vi "Unintentional Island Occurence.vi"(8 "error in":errorcluster, 10 "Unintentional Island":bool, 11 "SCADA in":refnum<class "EMS.lvclass">) -> (0 "error out":errorcluster, 3 "SCADA out":refnum<class "EMS.lvclass">)   [LabVIEW 2018, in "EMS Core.lvlib" / "EMS.lvclass"]
uses:
  EMS.lvclass
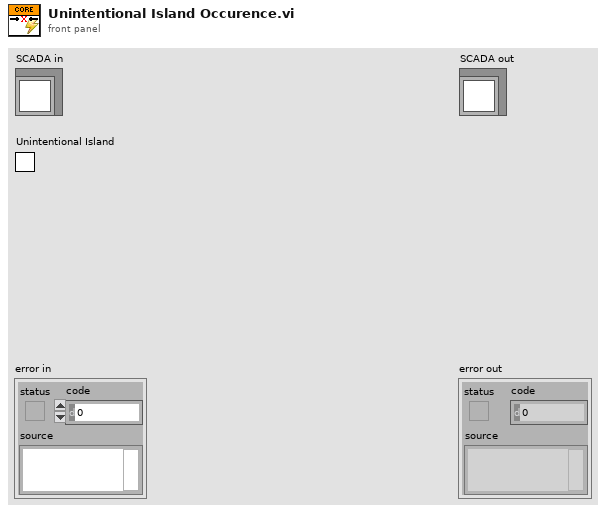
[diagram p1: front panel]
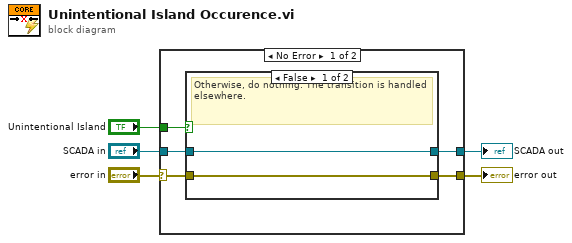
[diagram p0: block diagram]
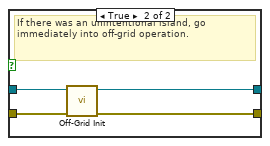
[diagram p2: hidden frame]
diagram:
  n1 = case shown="No Error" "error in" {
    selector: "error in" -> [w7 w18]
    tunnel: [w6 w18] -> w4
    tunnel: [w8 w17] -> w2
    tunnel: "SCADA in" -> [w9 w17]
    tunnel: "Unintentional Island" -> [w10 _]
    frame No Error {
      n2 = case shown="False" w10 {
        tunnel: w9 -> [w12 w16]
        tunnel: [w12 w15] -> w8
        tunnel: w7 -> [w11 w14]
        tunnel: [w11 w13] -> w6
        frame False {
          # "Otherwise, do nothing. The transition is handled elsewhere."
        }
        frame True {
          # "If there was an unintentional island, go immediately into off-grid operation."
          n3 = call "Off-Grid Init.vi"("error in"=w14, "SCADA in"=w16) -> ("error out"=w13:errorcluster, "SCADA out"=w15:refnum<class "EMS.lvclass">)  [unwired: 8 in]
        }
      }
    }
    frame Error {
    }
  }
  "error out" <- w4
  "SCADA out" <- w2
